vi "Send ActorsRef Container to All Actors.vi"(8 "error in (no error)":errorcluster, 11 "Core in":refnum<class "Core.lvclass">) -> (0 "error out":errorcluster, 3 "Core out":refnum<class "Core.lvclass">)   [LabVIEW 2019, in "Core.lvlib" / "Core.lvclass"]
uses:
  Core.lvclass
  C:/Projekty/_Wewnetrzne/PC_ActorFramework/07_Program/LABVIEW/02_Source/Modules/ModuleAbstract/ModuleAbstract.lvclass
  ModuleAbstract/ModuleAbstract.lvclass/ModuleAbstract.ctl
  Containers/ActorRefContainer/ActorRefContainer.lvclass/ActorRefContainer.ctl
  Containers/ActorRefContainer/Accessors/ActorRefContainer Read Modules.vi
  Containers/ActorRefContainer/Accessors/ActorRefContainer Read Logs.vi
  <vilib>/ActorFramework/Message Enqueuer/Message Enqueuer.lvclass
  ModuleAbstract/ModuleAbstract.lvclass
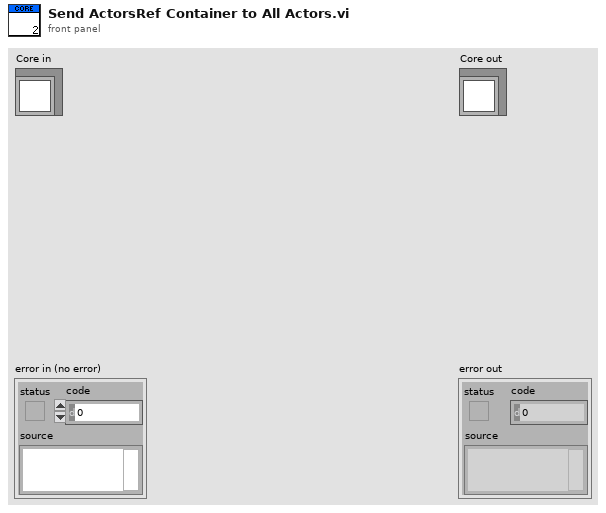
[diagram p1: front panel]
types:
  T1 = cluster{"Core":cluster{"ModRef":refnum<class "Message Enqueuer.lvclass">, "UIRef":refnum<class "Message Enqueuer.lvclass">}}
  T2 = cluster{"EventLog":cluster{"ModRef":refnum<class "Message Enqueuer.lvclass">, "UIRef":refnum<class "Message Enqueuer.lvclass">}}
  T3 = cluster{"ModRef":refnum<class "Message Enqueuer.lvclass">, "UIRef":refnum<class "Message Enqueuer.lvclass">}[]
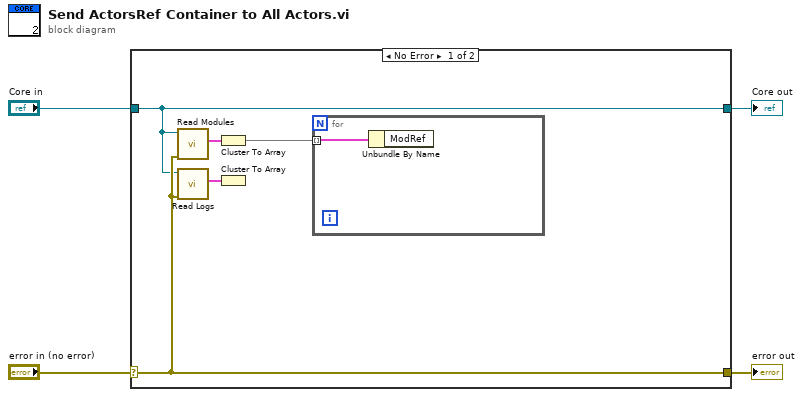
[diagram p0: block diagram]
diagram:
  n1 = case shown="No Error" "error in (no error)" {
    selector: "error in (no error)" -> [w9 w12]
    tunnel: [w9 w12] -> w3
    tunnel: [w6 w11] -> w1
    tunnel: "Core in" -> [w6 w11]
    frame No Error {
      n2 = call "Read Modules.vi"("error in (no error)"=w9, "ModuleAbstract in"=w6) -> ("Modules"=w8:T1)  [unwired: 7 in, 2 out]
      n3 = call "Read Logs.vi"("error in (no error)"=w9, "ModuleAbstract in"=w6) -> ("Logs"=w7:T2)  [unwired: 7 in, 2 out]
      n4 = Cluster To Array(cluster=w8) -> (array=w5:T3)
      n5 = Cluster To Array(cluster=w7) -> ()  [unwired: 1 out]
      n6 = for {
        tunnel: w5 -> [w10] mode=indexing
        n7 = Unbundle By Name(w10) -> ()  [unwired: 1 out]
      }
    }
    frame Error {
    }
  }
  "error out" <- w3
  "Core out" <- w1
